vi "SetSurfacePixels.vi"(8 "No Error":errorcluster, 10 "Pixels":u8[](array[numeric]) format="%.0x", 11 "Surface [SDL_Surface *]":i64) -> (0 "error out":errorcluster)   [LabVIEW 2026, in "SDL3.lvlib" / "Surface.lvlib"]
doc: "<B>Summary</B>\nSet surface pixels. Surface size won't change, meaning that excess pixels will be ignored."
uses:
  Surface.lvlib
  SurfaceFlags--ring.ctl
  Pixels/PixelFormat--enum.ctl
  Error/GetError-AnyThread.vi
  LV-Utilities/PointerSize.vi
  LV-Utilities/IsNULL.vi
  Pixels/U32ToPixelFormatEnum.vi
  <vilib>/Utility/error.llb/Error Cluster From Error Code.vi
  LV-Utilities/LV-Utilities.lvlib
  Pixels/Pixels.lvlib
panel:
  out "Surface Info":T3 {"flag" items=["SDL_SURFACE_PREALLOCATED"=1, "SDL_SURFACE_LOCK_NEEDED"=2, "SDL_SURFACE_LOCKED"=4, "SDL_SURFACE_SIMD_ALIGNED"=8]}
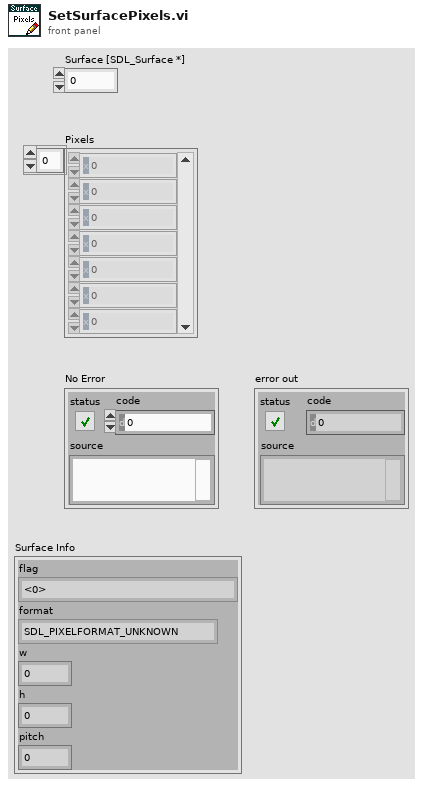
[diagram p1: front panel]
types:
  T1 = typedef "SDL3.lvlib/Surface.lvlib/SurfaceFlags--ring.ctl" = u32
  T2 = typedef "SDL3.lvlib/Pixels.lvlib/PixelFormat--enum.ctl" = enum32{"SDL_PIXELFORMAT_UNKNOWN", "SDL_PIXELFORMAT_INDEX1LSB", "SDL_PIXELFORMAT_INDEX1MSB", "SDL_PIXELFORMAT_INDEX2LSB", "SDL_PIXELFORMAT_INDEX2MSB", "SDL_PIXELFORMAT_INDEX4LSB", "SDL_PIXELFORMAT_INDEX4MSB", "SDL_PIXELFORMAT_INDEX8", "SDL_PIXELFORMAT_RGB332", "SDL_PIXELFORMAT_XRGB4444", "SDL_PIXELFORMAT_XBGR4444", "SDL_PIXELFORMAT_XRGB1555", "SDL_PIXELFORMAT_XBGR1555", "SDL_PIXELFORMAT_ARGB4444", "SDL_PIXELFORMAT_RGBA4444", "SDL_PIXELFORMAT_ABGR4444", "SDL_PIXELFORMAT_BGRA4444", "SDL_PIXELFORMAT_ARGB1555", "SDL_PIXELFORMAT_RGBA5551", "SDL_PIXELFORMAT_ABGR1555", "SDL_PIXELFORMAT_BGRA5551", "SDL_PIXELFORMAT_RGB565", "SDL_PIXELFORMAT_BGR565", "SDL_PIXELFORMAT_RGB24", "SDL_PIXELFORMAT_BGR24", "SDL_PIXELFORMAT_XRGB8888", "SDL_PIXELFORMAT_RGBX8888", "SDL_PIXELFORMAT_XBGR8888", "SDL_PIXELFORMAT_BGRX8888", "SDL_PIXELFORMAT_ARGB8888", "SDL_PIXELFORMAT_RGBA8888", "SDL_PIXELFORMAT_ABGR8888", "SDL_PIXELFORMAT_BGRA8888", "SDL_PIXELFORMAT_XRGB2101010", "SDL_PIXELFORMAT_XBGR2101010", "SDL_PIXELFORMAT_ARGB2101010", "SDL_PIXELFORMAT_ABGR2101010", "SDL_PIXELFORMAT_RGB48", "SDL_PIXELFORMAT_BGR48", "SDL_PIXELFORMAT_RGBA64", "SDL_PIXELFORMAT_ARGB64", "SDL_PIXELFORMAT_BGRA64", "SDL_PIXELFORMAT_ABGR64", "SDL_PIXELFORMAT_RGB48_FLOAT", "SDL_PIXELFORMAT_BGR48_FLOAT", "SDL_PIXELFORMAT_RGBA64_FLOAT", "SDL_PIXELFORMAT_ARGB64_FLOAT", "SDL_PIXELFORMAT_BGRA64_FLOAT", "SDL_PIXELFORMAT_ABGR64_FLOAT", "SDL_PIXELFORMAT_RGB96_FLOAT", "SDL_PIXELFORMAT_BGR96_FLOAT", "SDL_PIXELFORMAT_RGBA128_FLOAT", "SDL_PIXELFORMAT_ARGB128_FLOAT", "SDL_PIXELFORMAT_BGRA128_FLOAT", "SDL_PIXELFORMAT_ABGR128_FLOAT", "SDL_PIXELFORMAT_YV12", "SDL_PIXELFORMAT_IYUV", "SDL_PIXELFORMAT_YUY2", "SDL_PIXELFORMAT_UYVY", "SDL_PIXELFORMAT_YVYU", "SDL_PIXELFORMAT_NV12", "SDL_PIXELFORMAT_NV21", "SDL_PIXELFORMAT_P010", "SDL_PIXELFORMAT_EXTERNAL_OES"}
  T3 = cluster{"flag":T1, "format":T2, "w":i32, "h":i32, "pitch":i32}
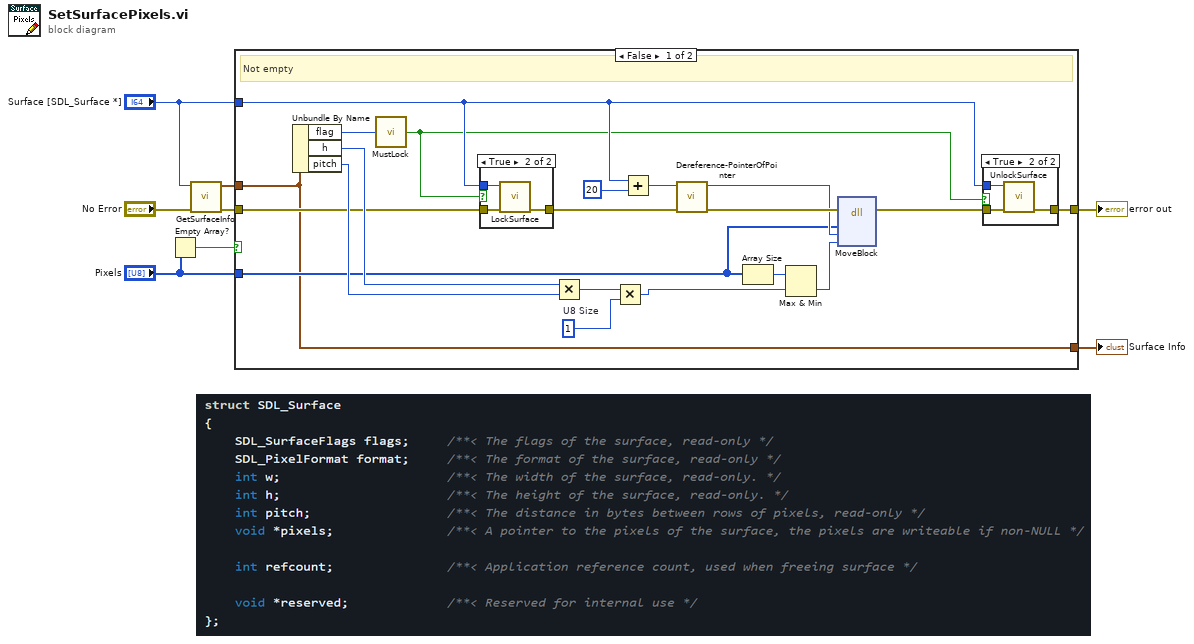
[diagram p0: block diagram]
diagram:
  n1 = Empty Array?(array="Pixels") -> (empty?=w3:bool)
  n2 = call "GetSurfaceInfo.vi"("No Error"="No Error", "Surface [SDL_Surface *]"="Surface [SDL_Surface *]") -> ("error out"=w2:errorcluster, "Surface Info"=w1:T3)  [unwired: 8 in]
  n3 = case shown="False" w3 {
    tunnel: [w24 w37] -> w7
    tunnel: "Surface [SDL_Surface *]" -> [w23 _]
    tunnel: [w9 w38] -> w5
    tunnel: "Pixels" -> [w14 _]
    tunnel: w2 -> [w10 w37]
    tunnel: w1 -> [w9 w38]
    frame False {
      w27 = 1  # U8 Size
      # "Not empty"
      n4 = Unbundle By Name(w9) -> ("flag"=w21:T1, "h"=w20:i32, "pitch"=w19:i32)
      n5 = call "MustLock.vi"("SurfaceFlags"=w21) -> ("Must Lock?"=w22:bool)
      n6 = case shown="True" w22 {
        tunnel: w10 -> [w29 w32]
        tunnel: [w29 w31] -> w18
        tunnel: w23 -> [_ w30]
        frame False {
        }
        frame True {
          n7 = call "LockSurface.vi"("No Error"=w32, "Surface [SDL_Surface *]"=w30) -> ("error out"=w31:errorcluster)  [unwired: 9 in]
        }
      }
      n8 = Multiply(x=w20, y=w19) -> (x*y=w26:i32)
      n9 = Multiply(x=w26, y=w27) -> (x*y=w12:i32)
      n10 = Add(x=w23, y=i64 20) -> (x+y=w16:i64)
      n11 = call "Dereference-PointerOfPointer.vi"("No Error"=w18, "Ptr of Ptr [void **]"=w16) -> ("error out"=w17:errorcluster, "Ptr [void *]"=w15:i64)  [unwired: 8 in]
      n12 = Array Size(array=w14) -> (size(s)=w13:i32)
      n13 = Max & Min(x=w13, y=w12) -> (min(x,y)=w11:i32)  [unwired: 1 out]
      n14 = dll-call lib="LabVIEW" fn="MoveBlock"(error in=w17, "Address"=w14, "Destination"=w15, "Size"=w11) -> (error out=w25:errorcluster)  [unwired: 6 in, 1 out]
      n15 = case shown="True" w22 {
        tunnel: w25 -> [w33 w36]
        tunnel: [w33 w35] -> w24
        tunnel: w23 -> [_ w34]
        frame False {
        }
        frame True {
          n16 = call "UnlockSurface.vi"("No Error"=w36, "Surface [SDL_Surface *]"=w34) -> ("error out"=w35:errorcluster)  [unwired: 9 in]
        }
      }
    }
    frame True {
      # "Empty"
    }
  }
  "error out" <- w7
  "Surface Info" <- w5
